vi "Draw Coord Line.vi"(8 "error in (no error)":errorcluster, 11 "GarphView in":refnum<class "GarphView.lvclass">) -> (0 "error out":errorcluster, 3 "GarphView out":refnum<class "GarphView.lvclass">)   [LabVIEW 2020, in "GarphView.lvlib" / "GarphView.lvclass"]
uses:
  GarphView.lvclass
  Coords Point.ctl
  <vilib>/Utility/miscctls.llb/LVPoint32TypeDef.ctl
  GarphView.lvclass/GarphView.ctl
  <vilib>/gpm_packages/@cs/lookup-table/Source/LookupTable/LookupTable.lvclass/LookupTable.ctl
  56d67af1-d11d-4c94-8f96-69c282d8b9f0.vi
  <vilib>/gpm_packages/@cs/lookup-table/Source/LookupTable/Read Table Reference.vi
  56d67af1-d11d-4c94-8f96-69c282d8b9f0.vi/527409de-c0d9-4f52-b5ac-fa7c64bbfe33.vi
  <vilib>/gpm_packages/@cs/lookup-table/Source/LookupTable/LookupTable.lvclass
panel:
  in  "XY":T1
  in  "Marker Options":T2={"Color"=16723218, "pen"={"Width"=2, "Style"=enum."Solid"}, "font"={"Font Name"="Arial", "Size"=26, "Strikeout?"=FALSE, "Italic?"=FALSE, "Underline?"=FALSE, "Outline?"=FALSE, "Shadow?"=FALSE, "Bold?"=TRUE, "FontColor"=393455}, "caption"=""}
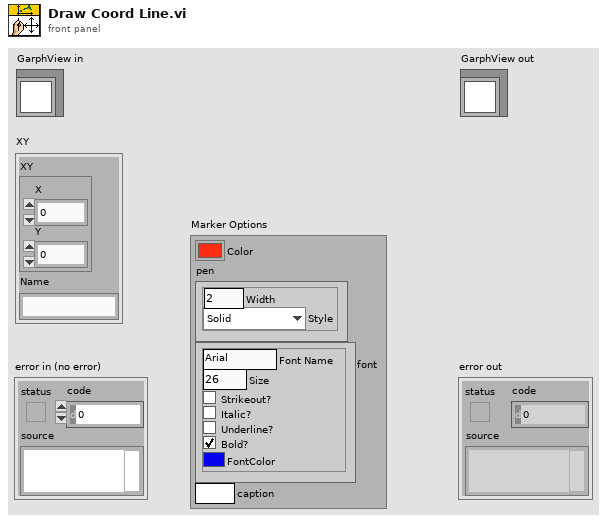
[diagram p1: front panel]
types:
  T1 = typedef "GarphView.lvlib/GarphView.lvclass/Coords Point.ctl" = cluster{"XY":cluster{"X":dbl, "Y":dbl}, "Name":string}
  T2 = cluster{"Color":u32, "pen":cluster{"Width":u16, "Style":enum32{"Solid", "Dash", "Dot", "DashDot", "DashDotDot"}}, "font":cluster{"Font Name":string, "Size":i16, "Strikeout?":bool, "Italic?":bool, "Underline?":bool, "Outline?":bool, "Shadow?":bool, "Bold?":bool, "FontColor":u32}, "caption":string}
  T3 = typedef "LVPoint32TypeDef.ctl" = cluster{"Horizontal":i32, "Vertical":i32}
  T4 = cluster{"Font Name:":string, "Size":i16, "Strikeout?":bool, "Italic?":bool, "Underline?":bool, "Outline?":bool, "Shadow?":bool, "Bold?":bool}
  T5 = enum16{"User-specified Font", "Application Font", "System Font", "Dialog Font"}
  T6 = cluster{"Width":u16, "Style":enum32{"Solid", "Dash", "Dot", "DashDot", "DashDotDot"}}
  T7 = cluster{"Font Name":string, "Size":i16, "Strikeout?":bool, "Italic?":bool, "Underline?":bool, "Outline?":bool, "Shadow?":bool, "Bold?":bool, "FontColor":u32}
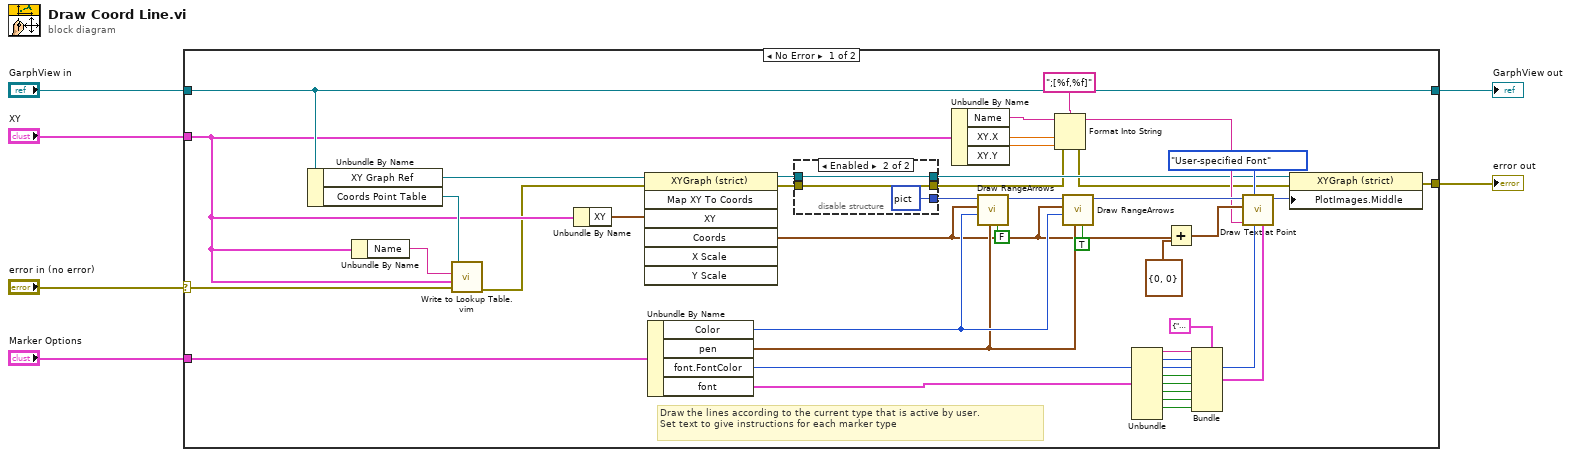
[diagram p0: block diagram]
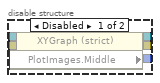
[diagram p2: hidden frame]
diagram:
  n1 = case shown="No Error" "error in (no error)" {
    selector: "error in (no error)" -> [w10 w60]
    tunnel: "Marker Options" -> [w47 _]
    tunnel: "GarphView in" -> [w16 w59]
    tunnel: "XY" -> [w8 _]
    tunnel: [w17 w60] -> w2
    tunnel: [w16 w59] -> w1
    frame No Error {
      # "Draw the lines according to the current type that is active by user.\nSet text to give instructions for each marker type"
      n2 = Unbundle By Name(w16) -> ("XY Graph Ref"=w26:refnum<vi>, "Coords Point Table"=w15:refnum<data-value>)
      n3 = Unbundle By Name(w8) -> ("Name"=w9:string)
      n4 = call "Write to Lookup Table.vim"("error in (no error)"=w10, "Item"=w8, "Item Name"=w9, "LookupTable Reference"=w15) -> ("error out"=w7:errorcluster)  [unwired: 5 in, 2 out]
      n5 = Unbundle By Name(w8) -> ("XY"=w14:cluster{"X":dbl, "Y":dbl})
      n6 = invoke class="XYGraph (strict)" method="Map XY To Coords"(reference=w26, error in=w7, "XY"=w14) -> (reference out=w24:refnum<vi>, error out=w23:errorcluster, "Coords"=w25:T3)  [unwired: 4 in, 4 out]
      n7 = Unbundle By Name(w47) -> ("Color"=w35:u32, "pen"=w34:T6, "font.FontColor"=w46:u32, "font"=w27:T7)
      n8 = disable-structure shown="Enabled" {
        disable-tunnel: w24 -> [w55 w57]
        disable-tunnel: w23 -> [w54 w56]
        disable-tunnel: [w53 picture data[5B] ("picture")] -> w22
        disable-tunnel: [w52 w57] -> w20
        disable-tunnel: [w51 w56] -> w19
        frame Disabled {
          n9 = property class="XYGraph (strict)"(reference=w55, error in=w54) -> (reference out=w52:refnum<vi>, error out=w51:errorcluster, "PlotImages.Middle"=w53:picture)
        }
        frame Enabled {
        }
      }
      n10 = Unbundle By Name(w8) -> ("Name"=w13:string, "XY.X"=w12:dbl, "XY.Y"=w11:dbl)
      n11 = call "Draw RangeArrows.vi"("Vertical"=FALSE, "pen"=w34, "Color"=w35, "position"=w25, "picture"=w22) -> ("new picture"=w29:picture)  [unwired: 6 in]
      n12 = Format Into String(format string=";[%f,%f]", initial string=w13, error in=w19, w12, w11) -> (resulting string=w31:string, error out=w18:errorcluster)
      n13 = call "Draw RangeArrows.vi"("Vertical"=TRUE, "pen"=w34, "Color"=w35, "position"=w25, "picture"=w29) -> ("new picture"=w49:picture)  [unwired: 6 in]
      n14 = Unbundle(w27) -> ("Font Name"=w44:string, "Size"=w43:i16, "Strikeout?"=w42:bool, "Italic?"=w41:bool, "Underline?"=w40:bool, "Outline?"=w39:bool, "Shadow?"=w38:bool, "Bold?"=w37:bool)  [unwired: 1 out]
      n15 = Add(x=w25, y=T3 {"Horizontal"=0, "Vertical"=0} ("x+y")) -> (x+y=w50:T3)
      n16 = Bundle(cluster=T4 {"Font Name:"="", "Size"=12, "Strikeout?"=FALSE, "Italic?"=FALSE, "Underline?"=FALSE, "Outline?"=FALSE, "Shadow?"=FALSE, "Bold?"=FALSE} ("[user-specified font]"), "Font Name:"=w44, "Size"=w43, "Strikeout?"=w42, "Italic?"=w41, "Underline?"=w40, "Outline?"=w39, "Shadow?"=w38, "Bold?"=w37) -> (w36:T4)
      n17 = call <vilib>:"Draw Text at Point.vi"("[user-specified font]"=w36, "text color(black)"=w46, "desired font(Application)"=T5."User-specified Font", "text"=w31, "origin"=w50, "picture"=w49) -> ("new picture"=w21:picture)  [unwired: 4 in, 1 out]
      n18 = property class="XYGraph (strict)"(reference=w20, error in=w18, "PlotImages.Middle"=w21) -> (error out=w17:errorcluster)  [unwired: 1 out]
    }
    frame Error {
    }
  }
  "error out" <- w2
  "GarphView out" <- w1
